vi "PCO_GetDoubleImageMode.vi"(8 "error in (no error)":errorcluster {"code" format="%x"}, 11 "ph":u64) -> (0 "error out":errorcluster {"code" format="%x"}, 1 "wDoubleImage":u16(ring) items=["OFF", "ON"], 2 "ErrorMessage":i32 format="%x", 3 "ph out":u64)   [LabVIEW 2019, in "SDK.lvlib" / "ImageSensor.lvlib"]
doc: "<b>Description:</b>\nThis function returns whether the camera is running in double image mode or not.\n\n<b>Supported camera type:</b>\nAll cameras\n\n<b>Descriptor dependency:</b>\nwDoubleImageDESC"
uses:
  ImageSensor.lvlib
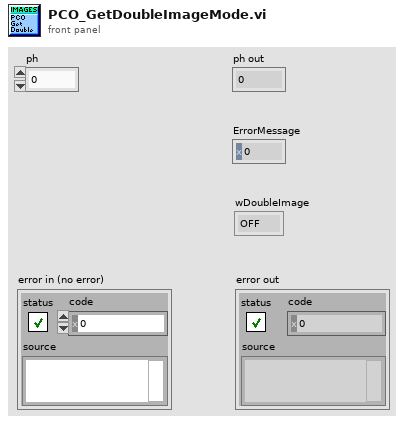
[diagram p1: front panel]
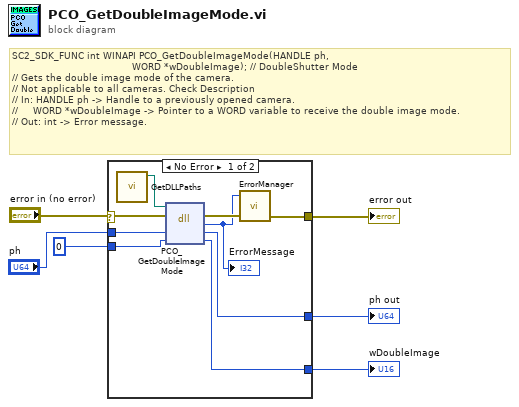
[diagram p0: block diagram]
diagram:
  # "SC2_SDK_FUNC int WINAPI PCO_GetDoubleImageMode(HANDLE ph,\n                                        WORD *wDoubleImage); // DoubleShutter Mode\n// Gets the double image mode of the camera.\n// Not applicable to all cameras. Check Description\n// In: HANDLE ph -> Handle to a previously opened camera.\n//     WORD *wDoubleImage -> Pointer to a WORD variable to receive the double image mode.\n// Out: int -> Error message."
  n1 = case shown="No Error" "error in (no error)" {
    selector: "error in (no error)" -> [w8 w18]
    tunnel: "ph" -> [w15 w17]
    tunnel: [w14 w17] -> w5
    tunnel: u16 0 ("wDoubleImage") -> [w13 w16]
    tunnel: [w12 w16] -> w3
    tunnel: [w10 w18] -> w2
    frame No Error {
      n2 = call "GetDLLPaths.vi"() -> ("SC2_Cam_Path"=w7:path)  [unwired: 8 in, 3 out]
      n3 = dll-call lib="?" fn="PCO_GetDoubleImageMode"(path in=w7, error in=w8, "ph"=w15, "wDoubleImage"=w13) -> (error out=w11:errorcluster, "return type"=w9:i32, "ph"=w14:u64, "wDoubleImage"=w12:u16)  [unwired: 1 in, 1 out]
      "ErrorMessage" <- w9
      n4 = call "ErrorManager.vi"("error in (no error)"=w11, "error code"=w9) -> ("error out"=w10:errorcluster)  [unwired: 2 in, 1 out]
    }
    frame Error {
    }
  }
  "ph out" <- w5
  "wDoubleImage" <- w3
  "error out" <- w2
